vi "Victor8246_Measure.vi"(8 "错误输入":errorcluster, 10 "读取命令":T1(ring), 11 "MyIndex":u8) -> (0 "错误输出":errorcluster, 1 "数值2":dbl, 2 "数值":dbl, 3 "返回状态":bool)   [LabVIEW 2015, in "Victor8246.lvlib"]
uses:
  Victor8246.lvlib
  <vilib>/Instr/_visa.llb/VISA Configure Serial Port (Instr).vi
panel:
  out "buff":string
  in  "记录编号":u8[](array[numeric]) format="%.0x"
  out "VISA资源":refnum<visa-resource-name>
  # "定时记录数据读取命令用到"
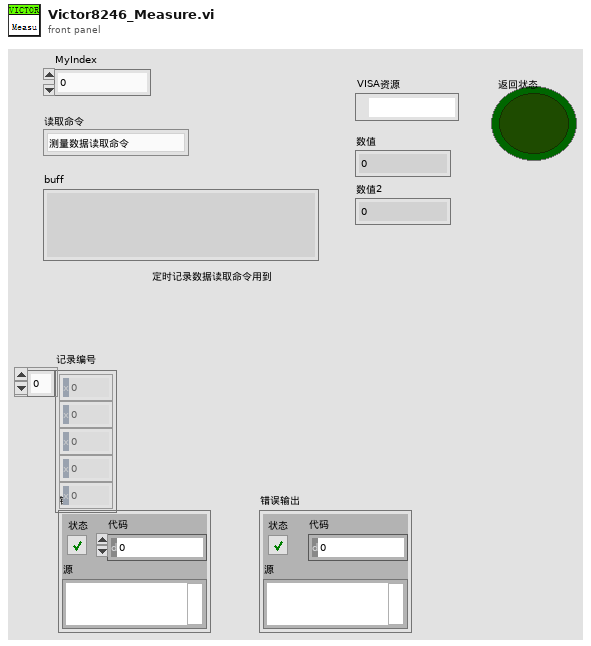
[diagram p1: front panel]
types:
  T1 = enum16{"测量数据读取命令", "测量工作状态读取命令", "定时记录配置读取命令", "定时记录数据读取命令"}
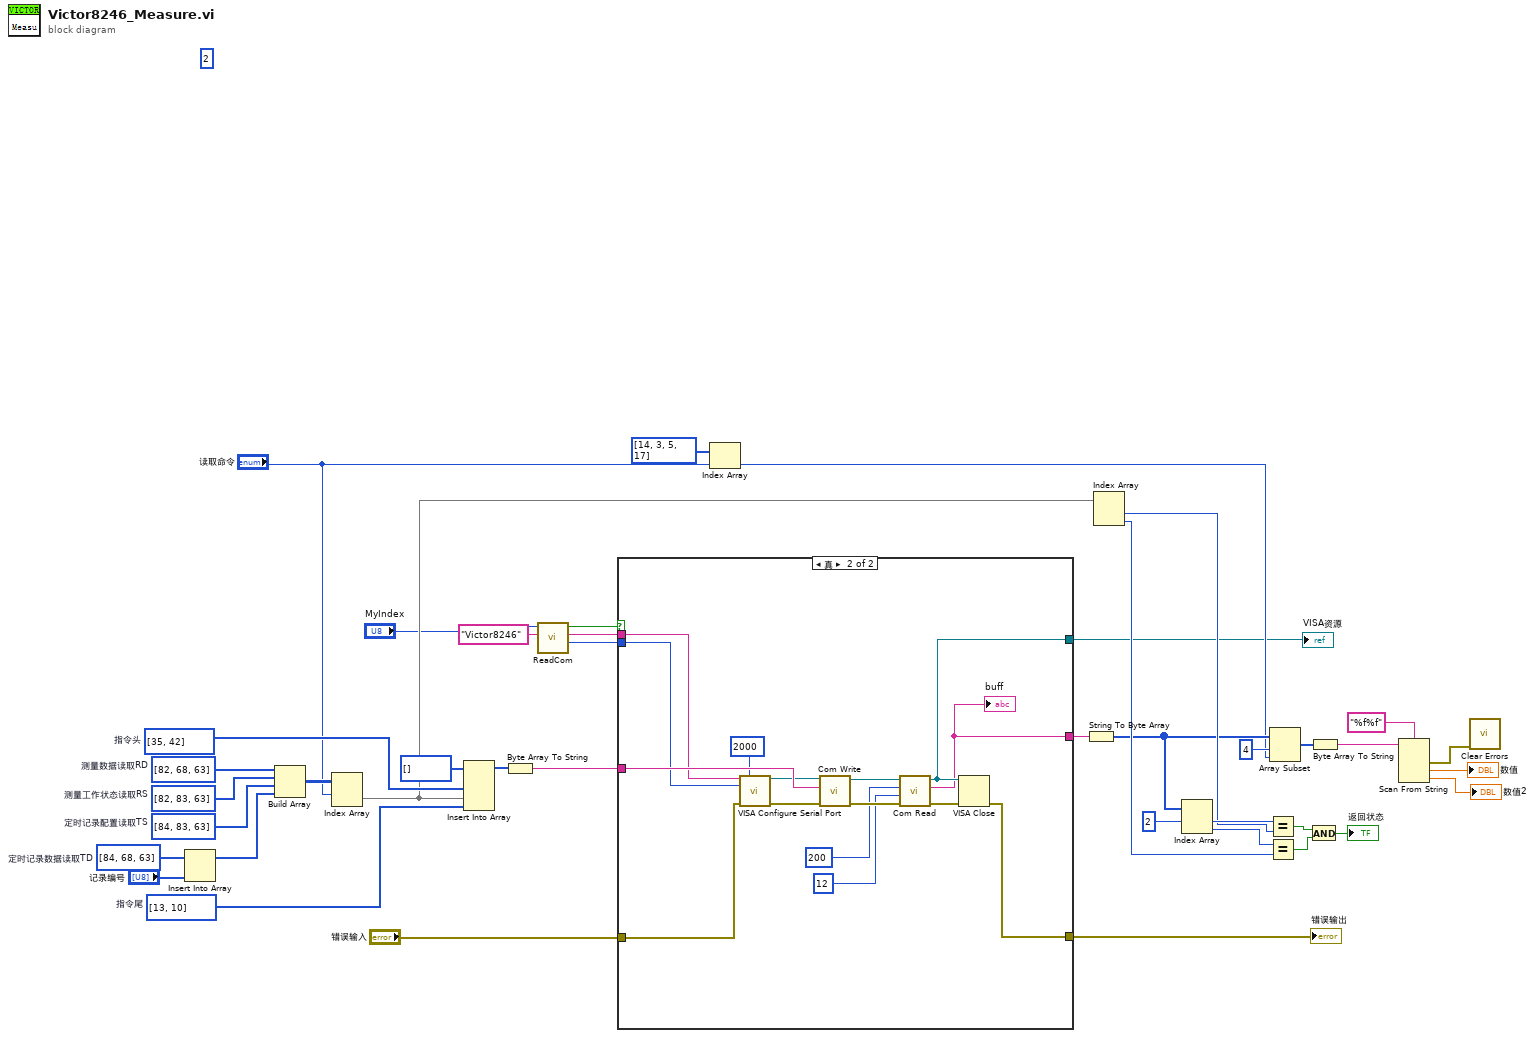
[diagram p0: block diagram]
diagram:
  w18 = u8[] [84, 68, 63]  # 定时记录数据读取TD
  w35 = u8[] [84, 83, 63]  # 定时记录配置读取TS
  w36 = u8[] [82, 83, 63]  # 测量工作状态读取RS
  w37 = u8[] [82, 68, 63]  # 测量数据读取RD
  w40 = u8[] [13, 10]  # 指令尾
  w41 = u8[] [35, 42]  # 指令头
  (unwired) 2
  n1 = Insert Into Array(array=w18, new element="记录编号") -> (w16:u8[])  [unwired: 1 in]
  n2 = Build Array(w37, w36, w35, w16) -> (w34:u8[][])
  n3 = Index Array(array=w34, index (row)="读取命令") -> (element=w27:u8[])  [unwired: 1 in]
  n4 = Insert Into Array(array=u8[] [] ("数组"), new element #1=w41, new element #2=w27, new element #3=w40) -> (w38:u8[])  [unwired: 1 in]
  n5 = Byte Array To String(unsigned byte array=w38) -> (string=w4:string)
  n6 = call "ReadCom.vi"("仪器名称"="Victor8246", "MyIndex"="MyIndex") -> ("Baudrate"=w6:i32, "COM"=w8:string, "OK?"=w7:bool)  [unwired: 7 in]
  n7 = case shown="真" w7 {
    tunnel: "错误输入" -> [_ w56]
    tunnel: w4 -> [_ w55]
    tunnel: w8 -> [_ w48]
    tunnel: w6 -> [_ w47]
    tunnel: [_ w44] -> w3
    tunnel: [_ w43] -> w2
    tunnel: [_ w42] -> w1
    frame False {
    }
    frame True {
      n8 = call-poly "VISA Configure Serial Port"("VISA resource name"=w48, "timeout (10sec)"=u32 2000, "baud rate (9600)"=w47, "error in (no error)"=w56) -> ("VISA resource name out"=w45:refnum<visa-resource-name>, "error out"=w49:errorcluster)  [unwired: 10 in]
      n9 = call "Com Write.vi"("错误输入（无错误）"=w49, "Wbuff"=w55, "VISA In"=w45) -> ("错误输出"=w54:errorcluster, "VISA Out"=w53:refnum<visa-resource-name>)  [unwired: 7 in]
      n10 = call "Com Read.vi"("错误输入（无错误）"=w54, "num"=u32 12, "超时"=u32 200, "VISA In"=w53) -> ("错误输出"=w50:errorcluster, "buff"=w42:string, "VISA Out"=w43:refnum<visa-resource-name>)  [unwired: 5 in]
      "buff" <- w42
      n11 = VISA Close(VISA resource name=w43, error in (no error)=w50) -> (error out=w44:errorcluster)
    }
  }
  "错误输出" <- w3
  "VISA资源" <- w2
  n12 = Index Array(array=i32[] [14, 3, 5, 17], index="读取命令") -> (element=w21:i32)
  n13 = String To Byte Array(string=w1) -> (unsigned byte array=w24:u8[])
  n14 = Index Array(array=w27) -> (element #1=w26:u8, element #2=w25:u8)  [unwired: 2 in]
  n15 = Index Array(array=w24, index #1=2 ("索引")) -> (element #1=w32:u8, element #2=w31:u8)  [unwired: 1 in]
  n16 = Equal?(x=w32, y=w26) -> (x = y?=w30:bool)
  n17 = Equal?(x=w31, y=w25) -> (x = y?=w29:bool)
  n18 = Array Subset(array=w24, index=4 ("索引"), length=w21) -> (w19:u8[])
  n19 = And(x=w30, y=w29) -> (x .and. y?=→"返回状态":bool)
  n20 = Byte Array To String(unsigned byte array=w19) -> (string=w14:string)
  n21 = Scan From String(format string="%f%f" ("格式字符串"), input string=w14) -> (error out=w11:errorcluster, output 1=→"数值":dbl, output 2=→"数值2":dbl)  [unwired: 4 in, 2 out]
  n22 = call <vilib>:"Clear Errors.vi"("error in (no error)"=w11) -> ()  [unwired: 5 in, 2 out]
